vi "CloseVS(Silent).vi"() -> ()   [LabVIEW 2011]
panel:
  in  "remote port":u16=2222
  in  "local port":u16=2221
  # "This VI sends a UDP message to the \nSilentVS.exe to close the VS Gateway"
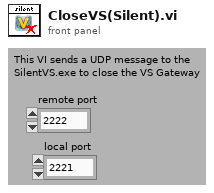
[diagram p1: front panel]
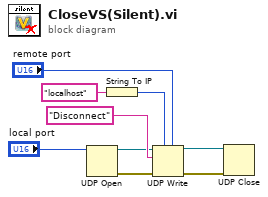
[diagram p0: block diagram]
diagram:
  n1 = UDP Open(11:"local port") -> (port=w4:refnum<k16>, 0:w3:errorcluster)  [unwired: 4 in, 1 out]
  n2 = String To IP(1:"localhost" ("name")) -> (0:w8:u32)
  n3 = UDP Write(address=w8, port or service name="remote port", connection ID=w4, data in="Disconnect", 8:w3) -> (error out=w5:errorcluster, 3:w6:refnum<k16>)  [unwired: 1 in]
  n4 = UDP Close(connection ID=w6, 8:w5) -> ()  [unwired: 2 out]
